vi "Read Offgrid VF Priority.vi"(8 "error in":errorcluster, 11 "EMS Generic in":refnum<class "EMS Generic.lvclass">) -> (0 "error out":errorcluster, 2 "Offgrid VF Priority":T1[](array[typedef]), 3 "EMS Generic out":refnum<class "EMS Generic.lvclass">)   [LabVIEW 2018, in "EMS Generic Actor.lvlib" / "EMS Generic.lvclass"]
uses:
  EMS Generic.lvclass
  <vilib>/ORNL/CSEISMIC DDS/CSEISMIC DDS Base/Data Types/Controls/DeviceID.ctl
  EMS Generic.lvclass/EMS Generic.ctl
  <vilib>/ORNL/CSEISMIC DDS/CSEISMIC DDS Base/CSEISMIC DDS.lvclass
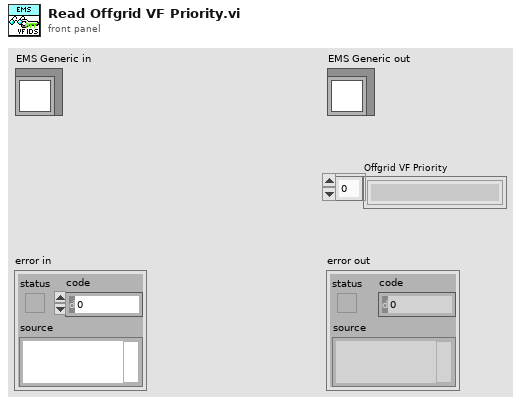
[diagram p1: front panel]
types:
  T1 = typedef "CSEISMIC DDS.lvlib/CSEISMIC DDS.lvclass/DeviceID.ctl" = string
  T2 = typedef "EMS Generic Actor.lvlib/EMS Generic.lvclass/Global Configuration.ctl" = cluster{"Microgrid ID":u8, "VF Device ID":T1, "Ongrid VF Priority":T1[], "Offgrid VF Priority":T1[], "AutoSwap Offgrid VF":u32, "AutoSwap Offgrid VF Delay (sec)":dbl, "AutoSwap Resynch VF":u32, "PCC Device ID":T1, "Device ID Array":T1[], "Nominal Voltage":dbl, "Nominal Frequency":dbl, "Resynch Timeout (sec)":dbl, "Island VF Activate Timeout (sec)":dbl, "Island PCC Target Power (kW)":dbl, "Island PCC Target Power Timeout (sec)":dbl, "Island Grid Settle Time (sec)":dbl, "Island PCC Failure Timeout (sec)":dbl, "Activation Devices Present Timeout (sec)":dbl, "Activation Devices Activated Timeout (sec)":dbl, "Blackstart VF GenMode Wait (sec)":dbl, "Blackstart VF DERCtrl Wait (sec)":dbl, "Blackstart Success Wait (sec)":dbl, "OnGrid Optimization Delay (sec)":dbl, "OffGrid Optimization Delay (sec)":dbl, "Resynch Frequency (Hz)":dbl, "Optimization Path":string}
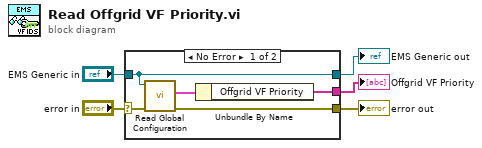
[diagram p0: block diagram]
diagram:
  n1 = case shown="No Error" "error in" {
    selector: "error in" -> [w9 w12]
    tunnel: [w6 w12] -> w4
    tunnel: [w10 w11] -> w2
    tunnel: "EMS Generic in" -> [w10 w11]
    tunnel: [w7 _] -> w1
    frame No Error {
      n2 = call "Read Global Configuration.vi"("error in"=w9, "EMS Generic in"=w10) -> ("error out"=w6:errorcluster, "Global Configuration"=w8:T2)  [unwired: 7 in, 1 out]
      n3 = Unbundle By Name(w8) -> ("Offgrid VF Priority"=w7:T1[])
    }
    frame Error {
    }
  }
  "error out" <- w4
  "EMS Generic out" <- w2
  "Offgrid VF Priority" <- w1
